vi "SetCommand.vi"(0 "Cypress CY8CKIT-059 in":refnum<class "Cypress CY8CKIT-059.lvclass">, 1 "Device Code":T2, 5 "Parameter 1":string, 7 "Parameter 2":string, 9 "Parameter 3":string, 11 "error in (no error)":errorcluster, 12 "Command Code":T1) -> (4 "Cypress CY8CKIT-059 out":refnum<class "Cypress CY8CKIT-059.lvclass">, 15 "error out":errorcluster)   [LabVIEW 2020, in "Cypress CY8CKIT-059.lvclass"]
doc: "It creats a command concatenating the given parameters. According to the device, it would send the command through the corresponding communication bus."
uses:
  Cypress CY8CKIT-059.lvclass
  Controls/Device Code.ctl
  Controls/Device Command Code.ctl
  Cypress CY8CKIT-059.lvclass/Cypress CY8CKIT-059.ctl
  Read Serial Port.vi
  Write Serial Port.vi
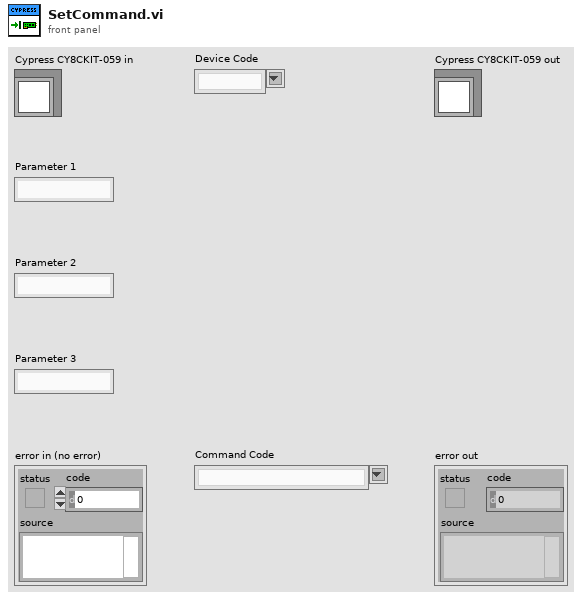
[diagram p1: front panel]
types:
  T1 = typedef "Device Command Code.ctl" = string
  T2 = typedef "Device Code.ctl" = string
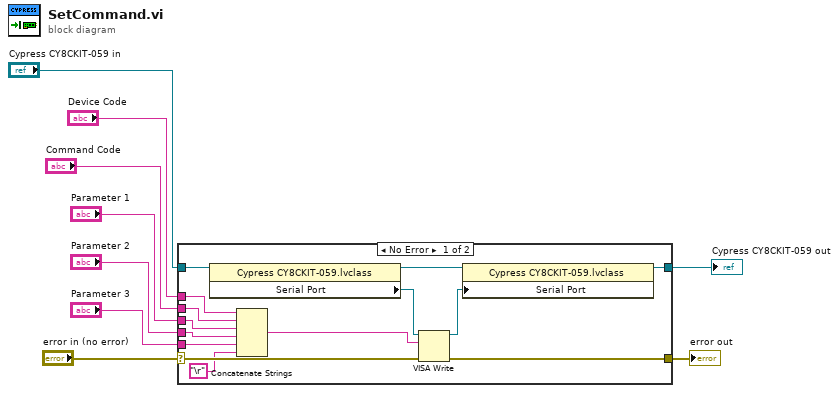
[diagram p0: block diagram]
diagram:
  n1 = case shown="No Error" "error in (no error)" {
    selector: "error in (no error)" -> [w14 w25]
    tunnel: "Device Code" -> [w23 _]
    tunnel: "Command Code" -> [w22 _]
    tunnel: "Parameter 1" -> [w21 _]
    tunnel: "Parameter 2" -> [w20 _]
    tunnel: "Parameter 3" -> [w19 _]
    tunnel: "Cypress CY8CKIT-059 in" -> [w18 w24]
    tunnel: [w12 w24] -> w3
    tunnel: [w13 w25] -> w1
    frame No Error {
      n2 = property class="Cypress CY8CKIT-059.lvclass"(reference=w18) -> (reference out=w17:refnum<class "Cypress CY8CKIT-059.lvclass">, "Serial Port"=w16:refnum<visa-resource-name>)  [unwired: 1 in, 1 out]
      n3 = Concatenate Strings(w23, w22, w21, w20, w19, "\r") -> (w15:string)
      n4 = VISA Write(VISA resource name=w16, write buffer=w15, error in (no error)=w14) -> (VISA resource name out=w11:refnum<visa-resource-name>, error out=w13:errorcluster)  [unwired: 1 out]
      n5 = property class="Cypress CY8CKIT-059.lvclass"(reference=w17, "Serial Port"=w11) -> (reference out=w12:refnum<class "Cypress CY8CKIT-059.lvclass">)  [unwired: 1 in, 1 out]
    }
    frame Error {
    }
  }
  "error out" <- w1
  "Cypress CY8CKIT-059 out" <- w3
